vi "Build Methods.vi"(6 "BuildType":T1 items=["simple", "Dialog", "PVUpdate", "Dialog&PV", "Asynch", "AsynchDial", "Ack"], 7 "ModifyDialog":bool=TRUE, 8 "error in (no error)":errorcluster, 9 "ProgressBarCluster":T2, 10 "Wiring Spec":T3, 11 "CS++Actor in":refnum<class "CS++Actor.lvclass">) -> (0 "error out":errorcluster, 3 "CS++Actor out":refnum<class "CS++Actor.lvclass">)   [LabVIEW 2016, in "CS++Actor.lvlib" / "CS++Actor.lvclass"]
doc: "Creates the methods for the new message."
uses:
  CS++Actor.lvclass
  CSPP_MessageMakerMain/BuildType.ctl
  CS++Actor.lvclass/CS++Actor.ctl
  CSPP_MessageMaker_Utilities/CS++MessagemakerUtilities.lvlib
  CSPP_MessageMakerMain/CS++MessageMakerMain.lvclass
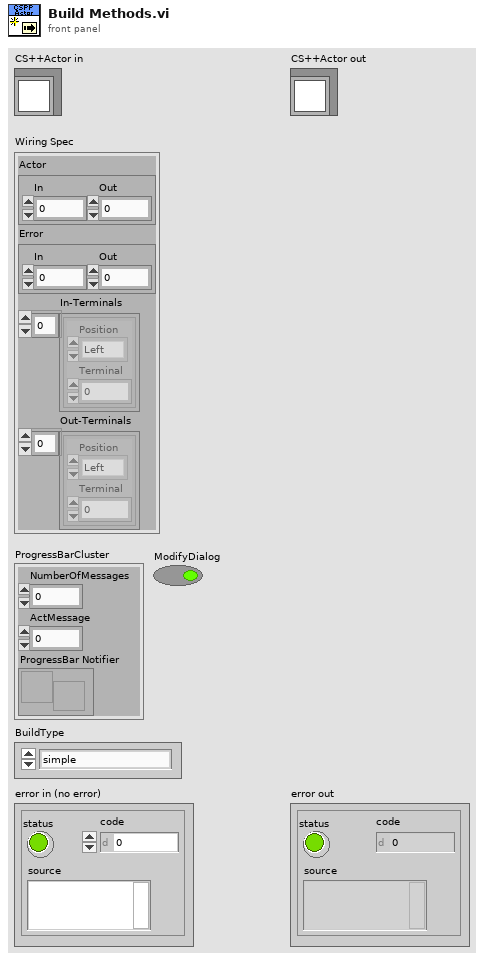
[diagram p1: front panel]
types:
  T1 = typedef "CS++MessageMakerMain.lvlib/CS++MessageMakerMain.lvclass/BuildType.ctl" = u16
  T2 = cluster{"NumberOfMessages":u16, "ActMessage":u16, "ProgressBar Notifier":refnum<notifier>}
  T3 = cluster{"Actor":cluster{"In":i32, "Out":i32}, "Error":cluster{"In":i32, "Out":i32}, "In-Terminals":cluster{"Position":enum16{"Left", "Top", "Bottom", "Right"}, "Terminal":i32}[], "Out-Terminals":cluster{"Position":enum16{"Left", "Top", "Bottom", "Right"}, "Terminal":i32}[]}
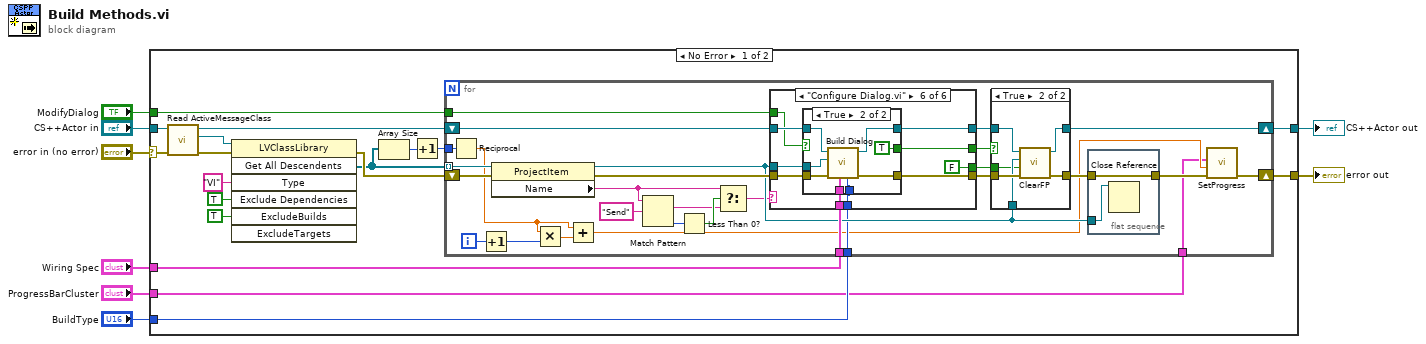
[diagram p0: block diagram]
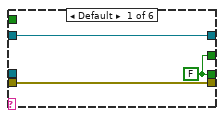
[diagram p3: hidden frame]
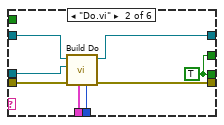
[diagram p4: hidden frame]
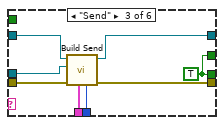
[diagram p5: hidden frame]
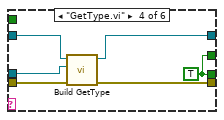
[diagram p6: hidden frame]
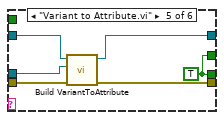
[diagram p7: hidden frame]
diagram:
  n1 = case shown="No Error" "error in (no error)" {
    selector: "error in (no error)" -> [w17 w118]
    tunnel: [w22 w118] -> w7
    tunnel: [w20 w117] -> w5
    tunnel: "CS++Actor in" -> [w18 w117]
    tunnel: "Wiring Spec" -> [w21 _]
    tunnel: "ProgressBarCluster" -> [w9 _]
    tunnel: "BuildType" -> [w14 _]
    tunnel: "ModifyDialog" -> [w13 _]
    frame No Error {
      n2 = call "Read ActiveMessageClass.vi"("error in (no error)"=w17, "CS++Actor in"=w18) -> ("error out"=w15:errorcluster, "ActiveMessageClass"=w19:refnum<vi>, "CS++Actor out"=w16:refnum<class "CS++Actor.lvclass">)  [unwired: 7 in]
      n3 = invoke class="LVClassLibrary" method="Get All Descendents"(reference=w19, error in=w15, "Type"="VI", "Exclude Dependencies"=TRUE ("ExcludeDependencies"), "ExcludeBuilds"=TRUE) -> (error out=w23:errorcluster, "All Descendents"=w12:refnum<vi>[])  [unwired: 2 in, 5 out]
      n4 = Array Size(array=w12) -> (size(s)=w11:i32)
      n5 = Increment(x=w11) -> (x+1=w10:i32)
      n6 = for {
        tunnel: w12 -> [w55] mode=indexing
        shift-right: [w30] -> w22
        shift-left: w23 -> [w54]
        tunnel: w21 -> [w52]
        shift-right: [w46] -> w20
        shift-left: w16 -> [w51]
        tunnel: w14 -> [w42]
        tunnel: w13 -> [w40]
        tunnel: w10 -> [w38]
        tunnel: w9 -> [w27]
        i -> [w50]
        n7 = Reciprocal(x=w38) -> (1/x=w37:dbl)
        n8 = Increment(x=w50) -> (x+1=w49:i32)
        n9 = property class="ProjectItem"(reference=w55, error in=w54) -> (reference out=w43:refnum<vi>, error out=w53:errorcluster, "Name"=w31:string)
        n10 = Multiply(x=w37, y=w49) -> (x*y=w48:dbl)
        n11 = Add(x=w37, y=w48) -> (x+y=w28:dbl)
        n12 = Match Pattern(string=w31, regular expression="Send") -> (match substring=w33:string, offset past match=w35:i32)  [unwired: 1 in, 2 out]
        n13 = Less Than 0?(x=w35) -> (x < 0?=w34:bool)
        n14 = Select(t=w31, s=w34, f=w33) -> (s? t:f=w32:string)
        n15 = case shown="\"Configure Dialog.vi\"" w32 {
          tunnel: [w68 w69 w77 w86 w92 w102] -> w47
          tunnel: w53 -> [w68 w76 w84 w90 w93 w106]
          tunnel: w43 -> [_ w73 w81 w87 w91 w103]
          tunnel: w52 -> [_ w75 w78 _ _ w99]
          tunnel: w51 -> [w67 w74 w83 w89 w95 w105]
          tunnel: [w67 w72 w82 w88 w94 w104] -> w45
          tunnel: w42 -> [_ w71 w79 _ _ w98]
          tunnel: [w66 w70 w80 w85 w96 FALSE] -> w41
          tunnel: w40 -> [_ _ _ _ _ w97]
          tunnel: [w66 w70 w80 w85 w96 w100] -> w39
          frame Default {
            w66 = FALSE
          }
          frame "Do.vi" {
            w70 = TRUE
            n16 = call "Build Do.vi"("BuildType"=w71, "Wiring Spec"=w75, "error in (no error)"=w76, "Do VI"=w73, "CS++Actor in"=w74) -> ("error out"=w69:errorcluster, "CS++Actor out"=w72:refnum<class "CS++Actor.lvclass">)  [unwired: 5 in]
          }
          frame "Send" {
            w80 = TRUE
            n17 = call "Build Send.vi"("BuildType"=w79, "Wiring Spec"=w78, "error in (no error)"=w84, "Send VI"=w81, "CS++Actor in"=w83) -> ("error out"=w77:errorcluster, "CS++Actor out"=w82:refnum<class "CS++Actor.lvclass">)  [unwired: 5 in]
          }
          frame "GetType.vi" {
            w85 = TRUE
            n18 = call "Build GetType.vi"("error in (no error)"=w90, "Get Type VI"=w87, "CS++Actor in"=w89) -> ("error out"=w86:errorcluster, "CS++Actor out"=w88:refnum<class "CS++Actor.lvclass">)  [unwired: 7 in]
          }
          frame "Variant to Attribute.vi" {
            w96 = TRUE
            n19 = call "Build VariantToAttribute.vi"("error in (no error)"=w93, "Get Type VI"=w91, "CS++Actor in"=w95) -> ("error out"=w92:errorcluster, "CS++Actor out"=w94:refnum<class "CS++Actor.lvclass">)  [unwired: 7 in]
          }
          frame "Configure Dialog.vi" {
            n20 = case shown="True" w97 {
              tunnel: w106 -> [w108 w116]
              tunnel: w105 -> [w107 w115]
              tunnel: [w107 w114] -> w104
              tunnel: w103 -> [_ w113]
              tunnel: [w108 w112] -> w102
              tunnel: [_ TRUE] -> w100
              tunnel: w99 -> [_ w110]
              tunnel: w98 -> [_ w109]
              frame False {
              }
              frame True {
                n21 = call "Build Dialog.vi"("BuildType"=w109, "Wiring Spec"=w110, "error in (no error)"=w116, "Dialog VI"=w113, "CS++Actor in"=w115) -> ("error out"=w112:errorcluster, "CS++Actor out"=w114:refnum<class "CS++Actor.lvclass">)  [unwired: 5 in]
              }
            }
          }
        }
        n22 = case shown="True" w39 {
          tunnel: w47 -> [w56 w63]
          tunnel: [w57 w62] -> w46
          tunnel: w45 -> [w57 w61]
          tunnel: [w56 w60] -> w44
          tunnel: w43 -> [_ w59]
          tunnel: w41 -> [_ w58]
          frame False {
          }
          frame True {
            n23 = call "ClearFP.vi"("error in (no error)"=w63, "ConPaneMode?"=w58, "ProjectItemRef"=w59, "CS++Actor in"=w61) -> ("error out"=w60:errorcluster, "CS++Actor out"=w62:refnum<class "CS++Actor.lvclass">)  [unwired: 6 in]
          }
        }
        n24 = flat-sequence {
          tunnel: [w65] -> w29
          tunnel: w44 -> [w65]
          tunnel: w43 -> [w64]
          frame #0 {
            n25 = Close Reference(reference=w64) -> ()  [unwired: 1 in, 1 out]
          }
        }
        n26 = call "SetProgress.vi"("error in (no error)"=w29, "SubStep"=w28, "ProgressBarCluster"=w27) -> ("error out"=w30:errorcluster)  [unwired: 8 in]
      }
    }
    frame Error {
    }
  }
  "error out" <- w7
  "CS++Actor out" <- w5
